vi "process_state_counts.vi"(11 "state-counts":u64[](array[numeric])=[0, 0, 0, 0, 0, 0]) -> (2 "State_times":dbl[](array[numeric]), 3 "Cs_time":dbl)   [LabVIEW 2017]
uses:
  controls/fpga_base_clock_constant.ctl
  controls/TsTicks_constant.ctl
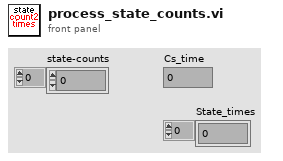
[diagram p1: front panel]
types:
  T1 = typedef "TsTicks_constant.ctl" = u32
  T2 = typedef "fpga_base_clock_constant.ctl" = u32
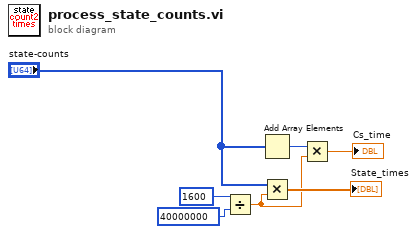
[diagram p0: block diagram]
diagram:
  n1 = Divide(x=T1 1600, y=T2 40000000) -> (x/y=w4:dbl)
  n2 = Add Array Elements(numeric array="state-counts") -> (sum=w3:u64)
  n3 = Multiply(x="state-counts", y=w4) -> (x*y=→"State_times":dbl[])
  n4 = Multiply(x=w3, y=w4) -> (x*y=→"Cs_time":dbl)
